vi "FirstLoad.vi"(6 "Downsample":i32, 7 "Cluster":T1, 8 "MessageBox":refnum<vi>, 9 "FileList":string[](array[string]), 10 "DEMP Folder":path) -> (1 "dt":dbl, 2 "Channels":string[](array[string]), 3 "DataPile":T2(array[cluster]), 4 "LoadedFiles":string[](array[string]), 5 "Keys":string[](array[string]))   [LabVIEW 2024]
uses:
  E:/CodeProjects/DEMPViewer/ClassLibrary1.dll
  ClassLibrary1.dll
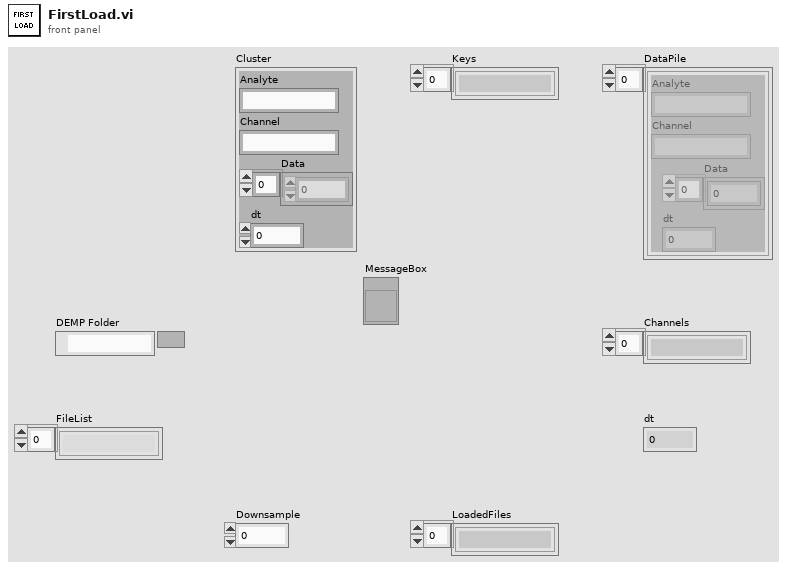
[diagram p1: front panel]
types:
  T1 = cluster{"Analyte":string, "Channel":string, "Data":dbl[], "dt":dbl}
  T2 = cluster{"Analyte":string, "Channel":string, "Data":dbl[], "dt":dbl}[]
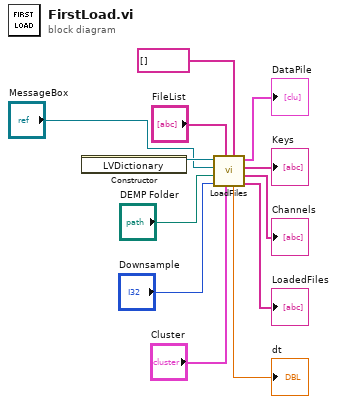
[diagram p0: block diagram]
diagram:
  n1 = constructor class="LVDictionary"() -> (reference out=w12:refnum<k24>)  [unwired: 3 in, 2 out]
  n2 = call "LoadFiles.vi"("FileListIn in"=string[] [], "Cluster"="Cluster", "FileList"="FileList", "Downsample"="Downsample", "DEMP Folder"="DEMP Folder", "MessageBox"="MessageBox", "FileDictionary"=w12) -> ("FileListIn out"=→"LoadedFiles":string[], "Channels"=→"Channels":string[], "Keys"=→"Keys":string[], "DataPile"=→"DataPile":T2, "dt"=→"dt":dbl)
